vi "U64 Tick Count.vi"(11 "error in (no error)":errorcluster) -> (8 "U64 Tick Count":u64, 15 "error out":errorcluster)   [LabVIEW 2018]
doc: "Creates a U64 version of the U32 mSec Timer Tick Count. Keeps track of wrapping."
uses:
  Instance           2 22Saved   U64 Tick Count .vi
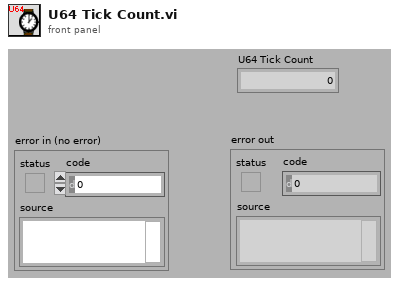
[diagram p1: front panel]
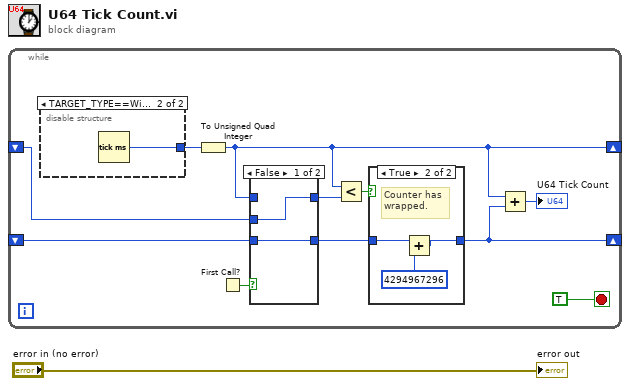
[diagram p0: block diagram]
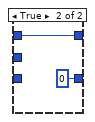
[diagram p3: hidden frame]
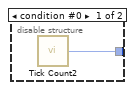
[diagram p4: hidden frame]
diagram:
  n1 = while {
    shift-right: [w4] -> _
    shift-left: _ -> [w2]
    shift-right: [w5] -> _
    shift-left: _ -> [w8]
    stop <- TRUE stop-if-true
    n2 = disable-structure shown="TARGET_TYPE==Windows" {
      disable-tunnel: [w21 w22] -> w7
      frame condition #0 {
        n3 = call "Tick Count2"() -> ("Tick Count(mSec)"=w21:u32)
      }
      frame condition #1 (active) {
        n4 = Tick Count (ms)() -> (millisecond timer value=w22:u32)
      }
    }
    n5 = To Unsigned Quad Integer(1:w7) -> (0:w4:u64)
    n6 = First Call?() -> (First Call?: T/F=w11:bool)
    n7 = case shown="False" w11 {
      tunnel: [w18 u64 0] -> w9
      tunnel: w8 -> [w18 _]
      tunnel: [w17 w19] -> w3
      tunnel: w4 -> [_ w19]
      tunnel: w2 -> [w17 _]
      frame False {
      }
      frame True {
      }
    }
    n8 = Less?(x=w4, y=w3) -> (x < y?=w10:bool)
    n9 = case shown="True" w10 {
      tunnel: w9 -> [w13 w16]
      tunnel: [w13 w15] -> w5
      frame False {
      }
      frame True {
        # "Counter has\nwrapped."
        n10 = Add(x=w16, y=u64 4294967296) -> (x+y=w15:u64)
      }
    }
    n11 = Add(x=w4, y=w5) -> (x+y=→"U64 Tick Count":u64)
  }
  "error out" <- "error in (no error)"
